vi "Delay pulse.vi"(10 "delay":u16, 11 "signal in":bool) -> (3 "delayed rising edge":bool)   [LabVIEW 2019, in "FPGA Utility.lvlib"]
uses:
  FPGA Utility.lvlib
  <instrlib>/_niInstr/Basic Elements/v1/FPGA/Private/Count Up U16.vi
  <instrlib>/_niInstr/Basic Elements/v1/FPGA/niInstr Basic Elements v1 FPGA.lvlib
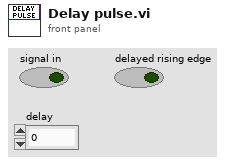
[diagram p1: front panel]
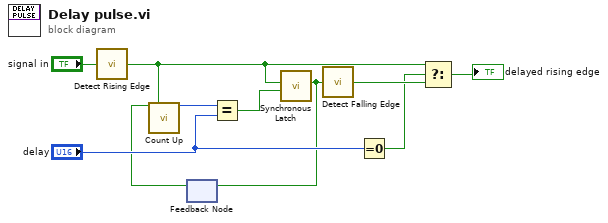
[diagram p0: block diagram]
diagram:
  n1 = call <instrlib>:"Detect Rising Edge.vi"("signal"="signal in") -> ("edge detected"=w3:bool)  [unwired: 14 in]
  n2 = feedback #1() -> (w1:bool)  [unwired: 1 in]
  n3 = call-poly <instrlib>:"Count Up.vi"("increment"=w1, "reset"=w3) -> ("count out"=w4:u16)  [unwired: 13 in]
  n4 = Equal?(x=w4, y="delay") -> (x = y?=w5:bool)
  n5 = call <instrlib>:"Synchronous Latch.vi"("clear"=w5, "set"=w3) -> ("out"=w2:bool)  [unwired: 9 in]
  n6 = feedback-in #1(w2) -> ()
  n7 = call <instrlib>:"Detect Falling Edge.vi"("signal"=w2) -> ("edge detected"=w8:bool)  [unwired: 14 in]
  n8 = Equal To 0?(x="delay") -> (x = 0?=w7:bool)
  n9 = Select(t=w3, s=w7, f=w8) -> (s? t:f=→"delayed rising edge":bool)
